vi "Destroy Event References.vi"(8 "error in (no error)":errorcluster, 11 "Actor-Events":T1) -> (0 "error out":errorcluster)   [LabVIEW 2018, in "Actor.lvlib" / "Actor.lvclass"]
uses:
  Actor.lvclass
  Event-References.ctl
  Stop.ctl
  Launched.ctl
  Actor-Interface.lvclass
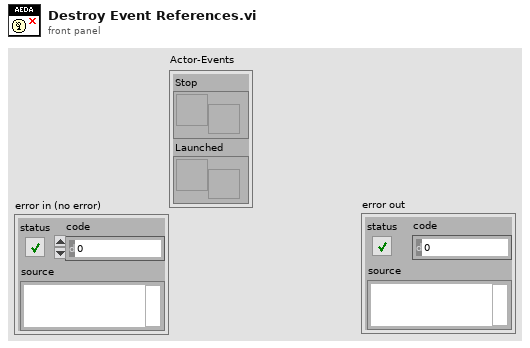
[diagram p1: front panel]
types:
  T1 = typedef "Actor.lvlib/Actor-Interface.lvclass/Event-References.ctl" = cluster{"Stop":refnum<user-event>, "Launched":refnum<user-event>}
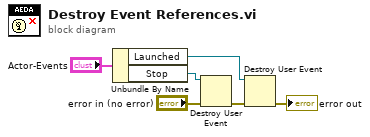
[diagram p0: block diagram]
diagram:
  n1 = Unbundle By Name("Actor-Events") -> ("Launched"=w3:refnum<user-event>, "Stop"=w5:refnum<user-event>)
  n2 = Destroy User Event(user event=w5, error in="error in (no error)") -> (error out=w2:errorcluster)
  n3 = Destroy User Event(user event=w3, error in=w2) -> (error out=→"error out":errorcluster)
